vi "Get Strain.vi"(6 "Channel":i32, 8 "error in (no error)":errorcluster, 11 "Instrument.Strain in":refnum<class "Instrument.Strain.lvclass">) -> (0 "error out":errorcluster, 2 "Strain (V)":dbl, 3 "Instrument.Strain out":refnum<class "Instrument.Strain.lvclass">)   [LabVIEW 2019, in "Instrument.Strain.lvclass"]
uses:
  Instrument.Strain.lvclass
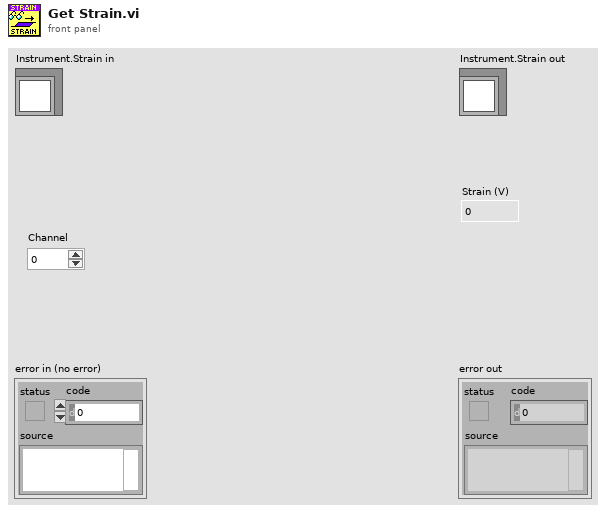
[diagram p1: front panel]
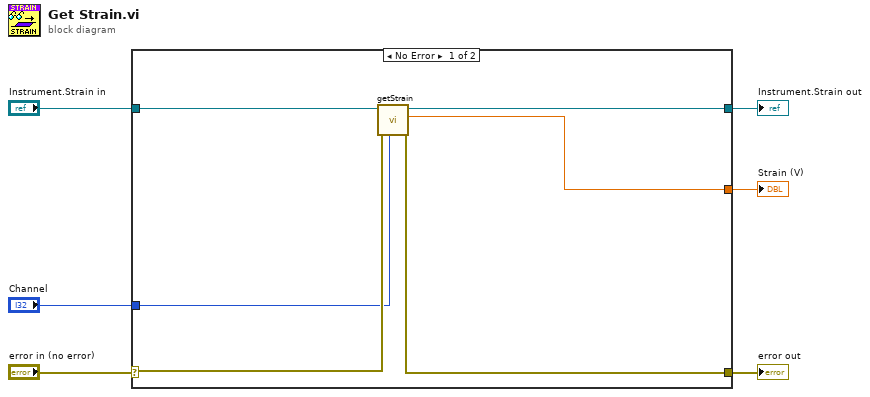
[diagram p0: block diagram]
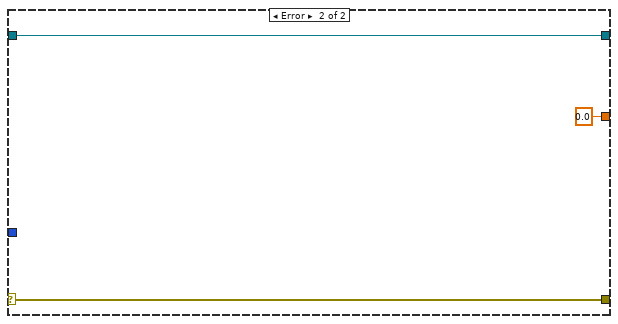
[diagram p2: hidden frame]
diagram:
  n1 = case shown="No Error" "error in (no error)" {
    selector: "error in (no error)" -> [w11 w15]
    tunnel: [w9 w15] -> w5
    tunnel: [w7 w14] -> w3
    tunnel: "Instrument.Strain in" -> [w12 w14]
    tunnel: "Channel" -> [w10 _]
    tunnel: [w8 0.0 ("Strain (V)")] -> w1
    frame No Error {
      n2 = call-dynamic "getStrain.vi"("Channel"=w10, "error in (no error)"=w11, "Instrument.Strain in"=w12) -> ("error out"=w9:errorcluster, "Strain (V)"=w8:dbl, "Instrument.Strain out"=w7:refnum<class "Instrument.Strain.lvclass">)  [unwired: 6 in]
    }
    frame Error {
    }
  }
  "error out" <- w5
  "Instrument.Strain out" <- w3
  "Strain (V)" <- w1
